vi "FGV_ChannelStatus.vi"(7 "Set":bool, 8 "error in (no error)":errorcluster caption="错误输入（无错误）", 10 "Index":i32, 11 "Start":bool) -> (0 "error out":errorcluster caption="错误输出", 3 "Start?":bool)   [LabVIEW 2018, in "CAN FD.lvlib"]
uses:
  CAN FD.lvlib
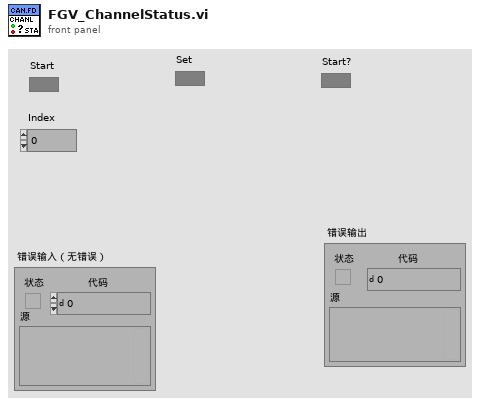
[diagram p1: front panel]
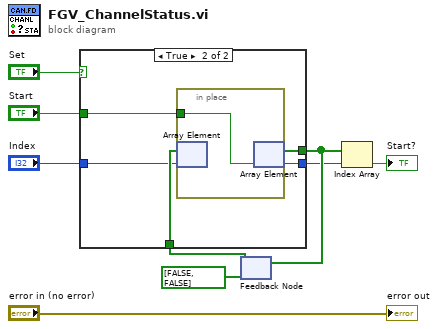
[diagram p0: block diagram]
diagram:
  n1 = feedback #1(bool[] [FALSE, FALSE]) -> (w6:bool[])
  n2 = case shown="True" "Set" {
    tunnel: "Start" -> [_ w13]
    tunnel: [w11 w14] -> w3
    tunnel: w6 -> [w11 w16]
    tunnel: "Index" -> [w10 w15]
    tunnel: [w10 w12] -> w2
    frame False {
    }
    frame True {
      n3 = in-place {
        in-place-border: w13 -> [w17]
        n4 = in-place-array #2(w16, w15) -> ()  [unwired: 1 out]
        n5 = in-place-array #2(w17) -> (w14:bool[], w12:i32)
      }
    }
  }
  n6 = feedback-in #1(w3) -> ()
  n7 = Index Array(array=w3, index=w2) -> (element=→"Start?":bool)
  "error out" <- "error in (no error)"
